vi "test template.vi"() -> (0 "error out":errorcluster)   [LabVIEW 2014, in "SQLite3LV Tests.lvlib"]
uses:
  SQLite3LV Tests.lvlib
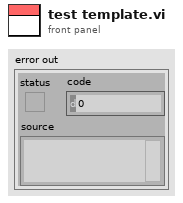
[diagram p1: front panel]
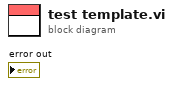
[diagram p0: block diagram]
diagram:
